vi "Write configuration.vi"(8 "error in":errorcluster, 10 "CEF Configuration":refnum<class "CEF_serializable configuration.lvclass">, 11 "Device Channel":refnum<class "Synchronization Channel.lvclass">) -> (0 "error out":errorcluster, 3 "Device Channel out":refnum<class "Synchronization Channel.lvclass">)   [LabVIEW 2025, in "Synchronization.lvlib" / "Synchronization Channel.lvclass"]
doc: "Copyright 2017 National Instruments Corporation\n\nLicensed under the Apache License, Version 2.0 (the \"License\"); you may not use this file except in compliance with the License. You may obtain a copy of the License at http://www.apache.org/licenses/LICENSE-2.0\nUnless required by applicable law or agreed to in writing, software distributed under the License is distributed on an \"AS IS\" BASIS, WITHOUT WARRANTIES OR CONDITIONS OF ANY KIND, either express or implied. See the License for the specific language governing permissions and limitations under the License."
uses:
  Synchronization Channel.lvclass
  Users/Public/Documents/Sandia National Labs/TSS Plugin/CEF.lvlibp/serializable configuration/CEF_serializable configuration.lvclass
  Synchronization Channel configuration/Synchronization Channel configuration.lvclass
  Synchronization Channel.lvclass/Synchronization Channel.ctl
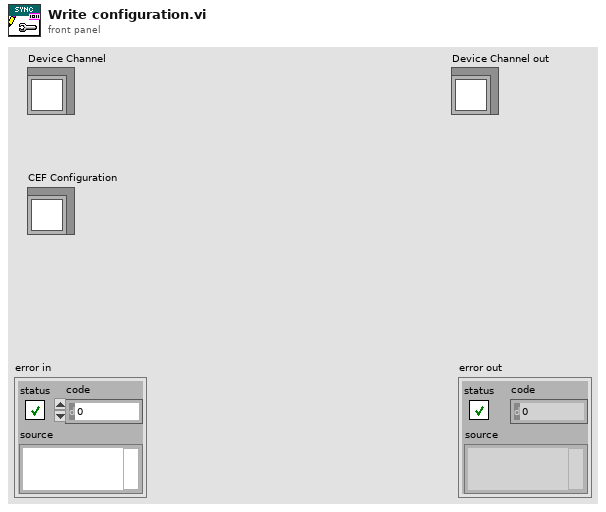
[diagram p1: front panel]
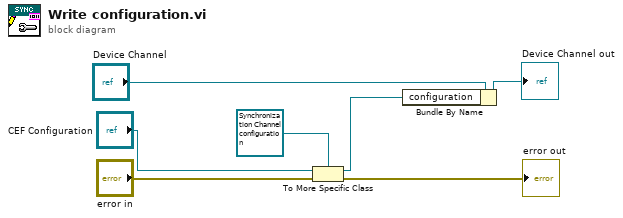
[diagram p0: block diagram]
diagram:
  n1 = To More Specific Class(target class=refnum<class "Synchronization Channel configuration.lvclass"> refnum ("configuration"), reference="CEF Configuration", error in="error in") -> (specific class reference=w4:refnum<class "Synchronization Channel configuration.lvclass">, error out=→"error out":errorcluster)
  n2 = Bundle By Name(cluster="Device Channel", "configuration"=w4) -> (→"Device Channel out":refnum<class "Synchronization Channel.lvclass">)
